vi "ReadInterleaved.vi"(7 "Poll Time (ms)":u32=10, 8 "error in":errorcluster, 9 "Timeout (s)":dbl=5.0, 10 "Samps Read per Chan":i32, 11 "Task in":refnum<class "WaveformTask.lvclass">) -> (0 "error out":errorcluster, 1 "Samples Remaining":u32, 2 "Data":sgl[](array[numeric]), 3 "Task out":refnum<class "WaveformTask.lvclass">)   [LabVIEW 2017, in "WaveformTask.lvclass"]
uses:
  WaveformTask.lvclass
  WaveformTask.lvclass/WaveformTask.ctl
  ErrorSelector.ctl
  <vilib>/rvi/errors/niLvFpgaAdjustHostInterfaceError.vi
  <vilib>/Utility/error.llb/Error Cluster From Error Code.vi
  DataFIFOs.ctl
  <vilib>/rvi/interface/nirviMethod/nirviMethod.xnode
  <vilib>/FPGAPlugInAG/Dynamic/niLvFpga_ReadFifo_Dynamic.vi
  <vilib>/rvi/errors/niLvFpgaMergeErrorWithErrorCode.vi
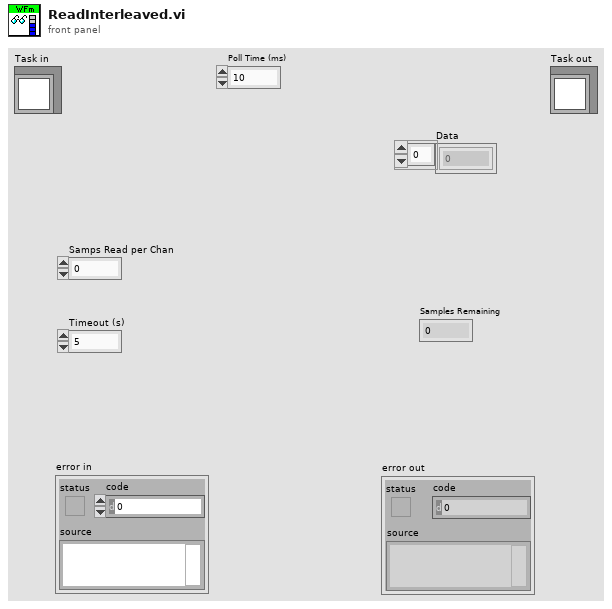
[diagram p1: front panel]
types:
  T1 = typedef "WaveformTask.lvclass/DataFIFOs.ctl" = refnum<k20>
  T2 = typedef "WaveformTask.lvclass/ErrorSelector.ctl" = enum16{"Read Timeout", "Module Underflow", "DMA Overflow", "Chan Count", "Run Timeout", "Start Timeout", "Stop Timeout"}
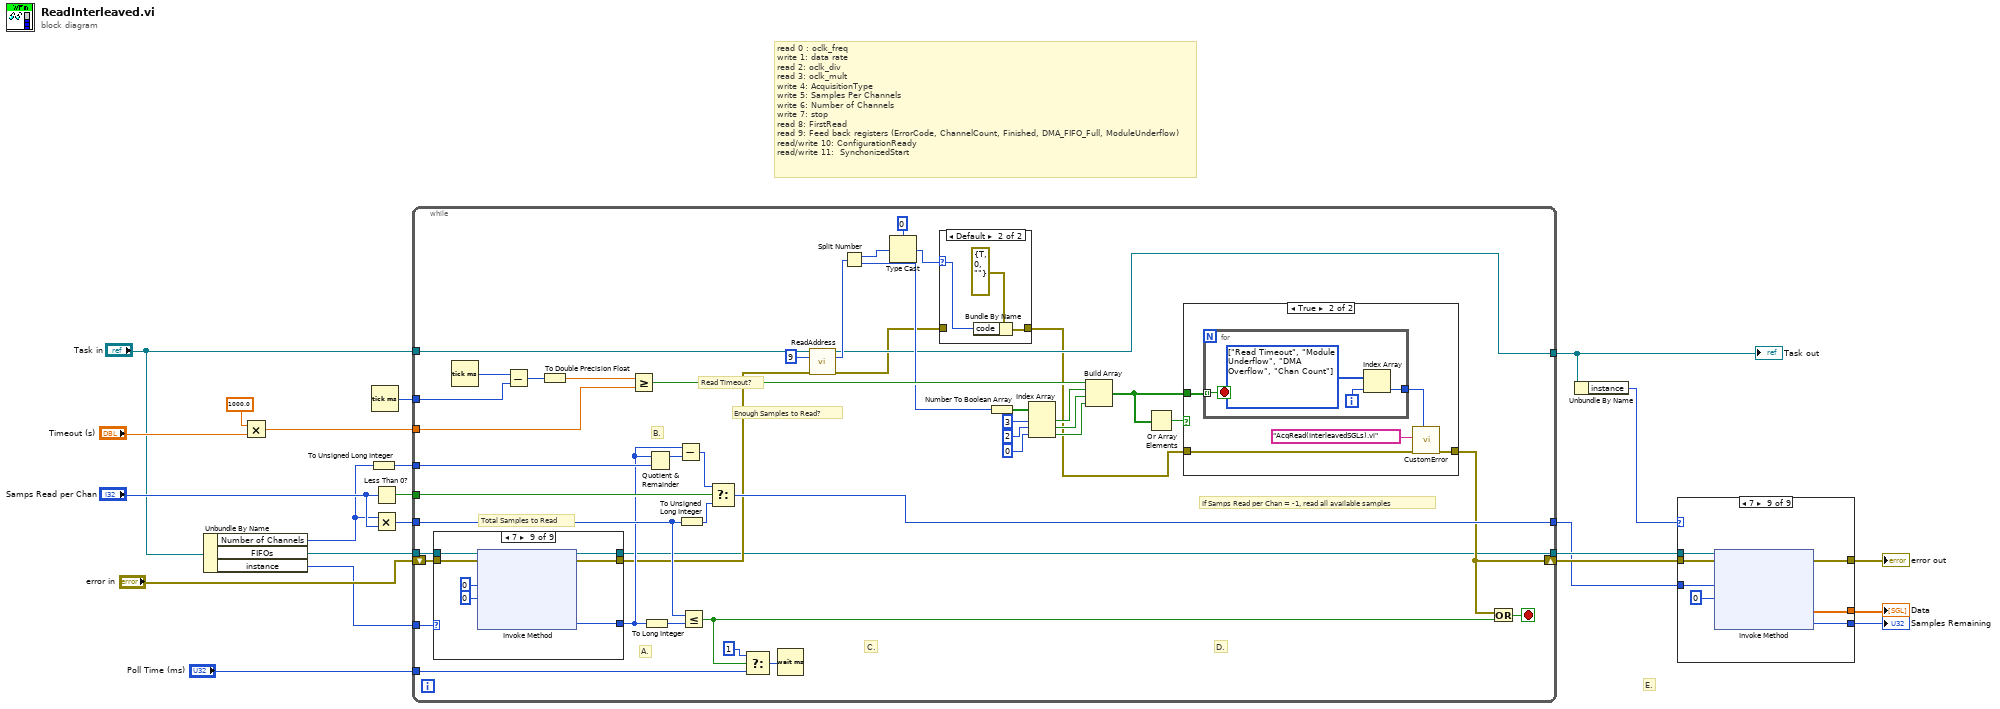
[diagram p0: block diagram]
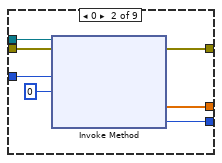
[diagram p3: hidden frame]
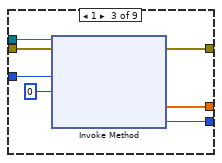
[diagram p4: hidden frame]
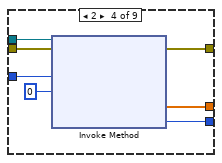
[diagram p5: hidden frame]
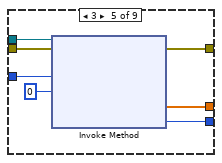
[diagram p6: hidden frame]
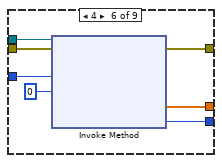
[diagram p7: hidden frame]
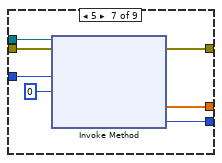
[diagram p8: hidden frame]
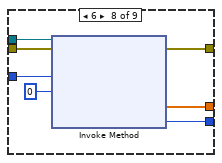
[diagram p9: hidden frame]
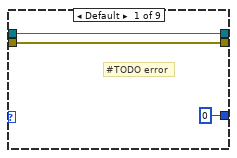
[diagram p11: hidden frame]
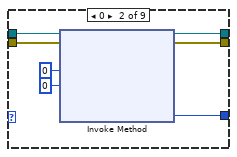
[diagram p12: hidden frame]
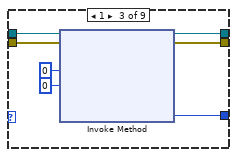
[diagram p13: hidden frame]
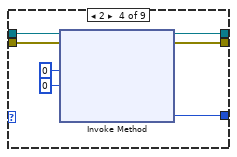
[diagram p14: hidden frame]
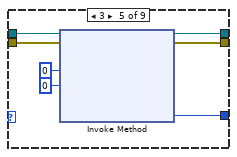
[diagram p15: hidden frame]
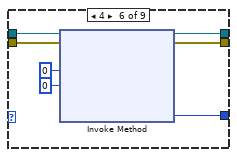
[diagram p16: hidden frame]
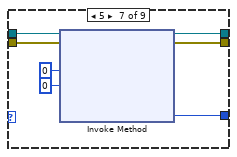
[diagram p17: hidden frame]
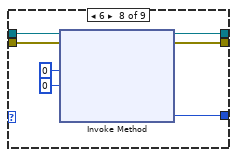
[diagram p18: hidden frame]
diagram:
  # "read 0 : oclk_freq\nwrite 1: data rate\nread 2: oclk_div\nread 3: oclk_mult\nwrite 4: AcquisitionType\nwrite 5: Samples Per Channels\nwrite 6: Number of Channels\nwrite 7: stop\nread 8: FirstRead\nread 9: Feed back registers (ErrorCode, ChannelCount, Finished, DMA_FIFO_Full, ModuleUnderflow)\nread/write 10: ConfigurationReady\nread/write 11:  SynchonizedStart"
  # "E."
  n1 = Unbundle By Name("Task in") -> ("Number of Channels"=w5:i32, "FIFOs"=w6:T1, "instance"=w3:u8)
  n2 = Multiply(x=1000.0 ("y"), y="Timeout (s)") -> (x*y=w19:dbl)
  n3 = To Unsigned Long Integer(number=w5) -> (unsigned 32bit integer=w13:u32)
  n4 = Tick Count (ms)() -> (millisecond timer value=w21:u32)
  n5 = Less Than 0?(x="Samps Read per Chan") -> (x < 0?=w15:bool)
  n6 = Multiply(x=w5, y="Samps Read per Chan") -> (x*y=w14:i32)
  n7 = while {
    tunnel: [w28] -> w17
    tunnel: w6 -> [w62]
    tunnel: w21 -> [w64]
    tunnel: w19 -> [w63]
    tunnel: "Poll Time (ms)" -> [w56]
    tunnel: [w49] -> w16
    tunnel: w14 -> [w51]
    tunnel: w15 -> [w52]
    tunnel: w13 -> [w53]
    shift-right: [w43] -> w18
    shift-left: "error in" -> [w61]
    tunnel: "Task in" -> [w42]
    tunnel: [w27] -> w2
    tunnel: w3 -> [w26]
    stop <- w67 stop-if-true
    # "A."
    # "D."
    # "C."
    # "B."
    # "If Samps Read per Chan = -1, read all available samples"
    # "Read Timeout?"
    # "Total Samples to Read"
    # "Enough Samples to Read?"
    n8 = case shown="7" w26 {
      tunnel: w62 -> [w74 w81 w88 w95 w102 w109 w116 w123 w130]
      tunnel: w61 -> [w73 w80 w87 w94 w101 w108 w115 w122 w129]
      tunnel: [u32 0 ("Elements Remaining") w77 w84 w91 w98 w105 w112 w119 w126] -> w46
      tunnel: [w73 w76 w83 w90 w97 w104 w111 w118 w125] -> w35
      tunnel: [w74 w75 w82 w89 w96 w103 w110 w117 w124] -> w28
      frame Default {
        # "#TODO error"
      }
      frame 0 {
        n9 = xnode "Invoke Method"("FPGA VI Reference In"=w81, "error in"=w80, "Number of Elements"=u32 0, "Timeout (ms)"=0) -> ("FPGA VI Reference Out"=w75:T1, "error out"=w76:errorcluster, "Elements Remaining"=w77:u32)  [unwired: 1 out]
      }
      frame 1 {
        n10 = xnode "Invoke Method"("FPGA VI Reference In"=w88, "error in"=w87, "Number of Elements"=u32 0, "Timeout (ms)"=0) -> ("FPGA VI Reference Out"=w82:T1, "error out"=w83:errorcluster, "Elements Remaining"=w84:u32)  [unwired: 1 out]
      }
      frame 2 {
        n11 = xnode "Invoke Method"("FPGA VI Reference In"=w95, "error in"=w94, "Number of Elements"=u32 0, "Timeout (ms)"=0) -> ("FPGA VI Reference Out"=w89:T1, "error out"=w90:errorcluster, "Elements Remaining"=w91:u32)  [unwired: 1 out]
      }
      frame 3 {
        n12 = xnode "Invoke Method"("FPGA VI Reference In"=w102, "error in"=w101, "Number of Elements"=u32 0, "Timeout (ms)"=0) -> ("FPGA VI Reference Out"=w96:T1, "error out"=w97:errorcluster, "Elements Remaining"=w98:u32)  [unwired: 1 out]
      }
      frame 4 {
        n13 = xnode "Invoke Method"("FPGA VI Reference In"=w109, "error in"=w108, "Number of Elements"=u32 0, "Timeout (ms)"=0) -> ("FPGA VI Reference Out"=w103:T1, "error out"=w104:errorcluster, "Elements Remaining"=w105:u32)  [unwired: 1 out]
      }
      frame 5 {
        n14 = xnode "Invoke Method"("FPGA VI Reference In"=w116, "error in"=w115, "Number of Elements"=u32 0, "Timeout (ms)"=0) -> ("FPGA VI Reference Out"=w110:T1, "error out"=w111:errorcluster, "Elements Remaining"=w112:u32)  [unwired: 1 out]
      }
      frame 6 {
        n15 = xnode "Invoke Method"("FPGA VI Reference In"=w123, "error in"=w122, "Number of Elements"=u32 0, "Timeout (ms)"=0) -> ("FPGA VI Reference Out"=w117:T1, "error out"=w118:errorcluster, "Elements Remaining"=w119:u32)  [unwired: 1 out]
      }
      frame 7 {
        n16 = xnode "Invoke Method"("FPGA VI Reference In"=w130, "error in"=w129, "Number of Elements"=u32 0, "Timeout (ms)"=0) -> ("FPGA VI Reference Out"=w124:T1, "error out"=w125:errorcluster, "Elements Remaining"=w126:u32)  [unwired: 1 out]
      }
    }
    n17 = Tick Count (ms)() -> (millisecond timer value=w60:u32)
    n18 = Subtract(x=w60, y=w64) -> (x-y=w66:u32)
    n19 = To Double Precision Float(number=w66) -> (double precision float=w65:dbl)
    n20 = Greater Or Equal?(x=w65, y=w63) -> (x >= y?=w59:bool)
    n21 = To Long Integer(number=w46) -> (32bit integer=w54:i32)
    n22 = Quotient & Remainder(x=w46, y=w53) -> (x-y*floor(x/y)=w48:u32)  [unwired: 1 out]
    n23 = Subtract(x=w46, y=w48) -> (x-y=w47:u32)
    n24 = To Unsigned Long Integer(number=w51) -> (unsigned 32bit integer=w50:u32)
    n25 = Less Or Equal?(x=w51, y=w54) -> (x <= y?=w57:bool)
    n26 = Select(t=w47, s=w52, f=w50) -> (s? t:f=w49:u32)
    n27 = Select(t=u32 1, s=w57, f=w56) -> (s? t:f=w58:u32)
    n28 = Wait (ms)(milliseconds to wait=w58) -> ()  [unwired: 1 out]
    n29 = call "ReadAddress.vi"("Task in"=w42, "address"=u64 9, "error in (no error)"=w35) -> ("Task out"=w27:refnum<class "WaveformTask.lvclass">, "data"=w40:u64, "error out"=w24:errorcluster)  [unwired: 10 in]
    n30 = Split Number(x=w40) -> (hi(x)=w39:u32, lo(x)=w37:u32)
    n31 = Type Cast(type=0, x=w39) -> (*(type *) &x=w25:i32)
    n32 = case shown="Default" w25 {
      selector: w25 -> [_ w70]
      tunnel: w24 -> [w68 _]
      tunnel: [w68 w69] -> w23
      frame 0 {
      }
      frame Default {
        n33 = Bundle By Name(cluster=errorcluster {"status"=TRUE, "code"=0, "source"=""} ("error out"), "code"=w70) -> (w69:errorcluster)
      }
    }
    n34 = Number To Boolean Array(number=w37) -> (Boolean array=w36:bool[])
    n35 = Index Array(array=w36, index #1=3 ("index"), index #2=2 ("index"), index #3=0 ("index")) -> (element #1=w31:bool, element #2=w30:bool, element #3=w29:bool)
    n36 = Build Array(w59, w31, w30, w29) -> (w44:bool[])
    n37 = Or Array Elements(Boolean array=w44) -> (logical OR=w45:bool)
    n38 = case shown="True" w45 {
      tunnel: [w131 w135] -> w43
      tunnel: w23 -> [w131 w136]
      tunnel: w44 -> [_ w134]
      frame False {
      }
      frame True {
        n39 = for {
          tunnel: w134 -> [w140] mode=indexing
          tunnel: [w138] -> w133
          i -> [w139]
          stop <- w140 stop-if-true
          w137 = T2[] [enum."Read Timeout", enum."Module Underflow", enum."DMA Overflow", enum."Chan Count"] items=["Read Timeout", "Module Underflow", "DMA Overflow", "Chan Count", "Run Timeout", "Start Timeout", "Stop Timeout"]
          n40 = Index Array(array=w137, index=w139) -> (element=w138:T2)
        }
        n41 = call "CustomError.vi"("Error Selector"=w133, "error in (no error)"=w136, "VI name"="AcqRead(InterleavedSGLs).vi" ("Calling VI")) -> ("error out"=w135:errorcluster)  [unwired: 8 in]
      }
    }
    n42 = Or(x=w43, y=w57) -> (x .or. y?=w67:bool)
  }
  "Task out" <- w2
  n43 = Unbundle By Name(w2) -> ("instance"=w1:u8)
  n44 = case shown="7" w1 {
    tunnel: [w141 w148 w155 w162 w169 w176 w183 w190 w197] -> w22
    tunnel: w18 -> [w141 w147 w154 w161 w168 w175 w182 w189 w196]
    tunnel: w17 -> [_ w146 w153 w160 w167 w174 w181 w188 w195]
    tunnel: w16 -> [_ w145 w152 w159 w166 w173 w180 w187 w194]
    tunnel: [_ w143 w150 w157 w164 w171 w178 w185 w192] -> w8
    tunnel: [_ w142 w149 w156 w163 w170 w177 w184 w191] -> w7
    frame Default {
      # "#TODO Error"
    }
    frame 0 {
      n45 = xnode "Invoke Method"("FPGA VI Reference In"=w146, "error in"=w147, "Number of Elements"=w145, "Timeout (ms)"=0) -> ("error out"=w148:errorcluster, "Data"=w143:sgl[], "Elements Remaining"=w142:u32)  [unwired: 1 out]
    }
    frame 1 {
      n46 = xnode "Invoke Method"("FPGA VI Reference In"=w153, "error in"=w154, "Number of Elements"=w152, "Timeout (ms)"=0) -> ("error out"=w155:errorcluster, "Data"=w150:sgl[], "Elements Remaining"=w149:u32)  [unwired: 1 out]
    }
    frame 2 {
      n47 = xnode "Invoke Method"("FPGA VI Reference In"=w160, "error in"=w161, "Number of Elements"=w159, "Timeout (ms)"=0) -> ("error out"=w162:errorcluster, "Data"=w157:sgl[], "Elements Remaining"=w156:u32)  [unwired: 1 out]
    }
    frame 3 {
      n48 = xnode "Invoke Method"("FPGA VI Reference In"=w167, "error in"=w168, "Number of Elements"=w166, "Timeout (ms)"=0) -> ("error out"=w169:errorcluster, "Data"=w164:sgl[], "Elements Remaining"=w163:u32)  [unwired: 1 out]
    }
    frame 4 {
      n49 = xnode "Invoke Method"("FPGA VI Reference In"=w174, "error in"=w175, "Number of Elements"=w173, "Timeout (ms)"=0) -> ("error out"=w176:errorcluster, "Data"=w171:sgl[], "Elements Remaining"=w170:u32)  [unwired: 1 out]
    }
    frame 5 {
      n50 = xnode "Invoke Method"("FPGA VI Reference In"=w181, "error in"=w182, "Number of Elements"=w180, "Timeout (ms)"=0) -> ("error out"=w183:errorcluster, "Data"=w178:sgl[], "Elements Remaining"=w177:u32)  [unwired: 1 out]
    }
    frame 6 {
      n51 = xnode "Invoke Method"("FPGA VI Reference In"=w188, "error in"=w189, "Number of Elements"=w187, "Timeout (ms)"=0) -> ("error out"=w190:errorcluster, "Data"=w185:sgl[], "Elements Remaining"=w184:u32)  [unwired: 1 out]
    }
    frame 7 {
      n52 = xnode "Invoke Method"("FPGA VI Reference In"=w195, "error in"=w196, "Number of Elements"=w194, "Timeout (ms)"=0) -> ("error out"=w197:errorcluster, "Data"=w192:sgl[], "Elements Remaining"=w191:u32)  [unwired: 1 out]
    }
  }
  "error out" <- w22
  "Data" <- w8
  "Samples Remaining" <- w7
